vi "LV to ITX 2D AutoPlot.vi"(0 "filename":string, 1 "path":path, 5 "Notes":string, 7 "2D Array":dbl[][](array[numeric]), 9 "X, Y Arrays":cluster{"X 1D Array":dbl[], "Y 1D Array":dbl[]}={"X 1D Array"=[0.0, 1.0], "Y 1D Array"=[0.0, 1.0]}, 11 "X, Y wavenames":string[](array[string])=["x_", "y_"], 12 "X,Y,Z Labels":string[](array[string])=["x", "y"]) -> (4 "file":path)   [LabVIEW 2011]
doc: "Write your 2D data to ITX file. This AutoPlot VI adds commands that will automatically create in Igor an intensity graph with X and Y axes scaled by the 1D arrays, allowing you to quickly view your data.\n\n-- path: base path to save data\n-- filename: base filename\n-- Notes: add any notes here to help you remember what experiment you did\n-- 2D Array: Intensity data\n-- X,Y Arrays: These are used to apply an appropriate scaling to the intensity graph\n-- X,Y wavenames: Default \"x_\" and \"y_\" are fine.\n-- X,Y,Z Labels: Labels for plotting in Igor."
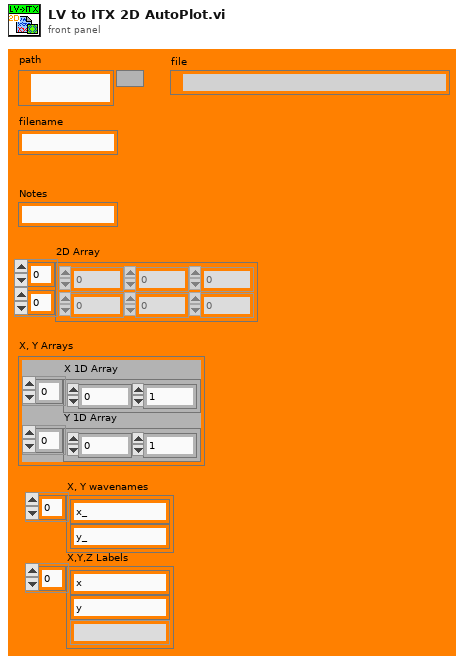
[diagram p1: front panel]
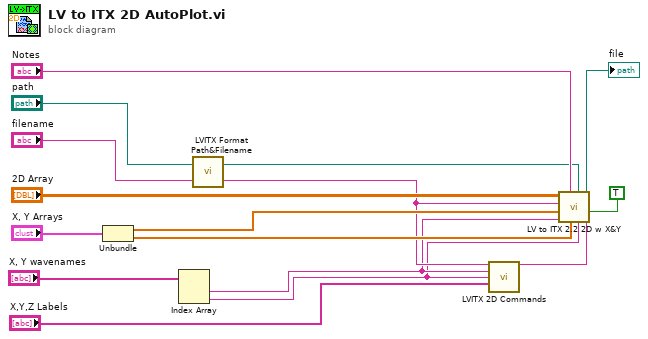
[diagram p0: block diagram]
diagram:
  n1 = Unbundle("X, Y Arrays") -> ("X 1D Array"=w10:dbl[], "Y 1D Array"=w9:dbl[])
  n2 = Index Array(array="X, Y wavenames") -> (element #1=w5:string, element #2=w4:string)  [unwired: 2 in]
  n3 = call "LVITX Format Path&Filename.vi"("filename"="filename", "path"="path") -> ("file name without extension"=w6:string, "dup file"=w11:path)
  n4 = call "LVITX 2D Commands.vi"("2D wavename"=w6, "X wavename"=w5, "Y wavename"=w4, "X,Y,Z Labels"="X,Y,Z Labels") -> ("result string"=w12:string)  [unwired: 2 in, 9 out]
  n5 = call "LV to ITX 2.2 2D w X&Y.vi"("Commands"=w12, "Kill X&Y waves?"=TRUE, "Y Array name"=w4, "filename"=w11, "Y 1D Array"=w9, "Notes"="Notes", "X  Array name"=w5, "X 1D Array"=w10, "2D Array name"=w6, "2D Array"="2D Array") -> ("file"=→"file":path)  [unwired: 1 out]
